vi "PathPlanner_PathPlanner_CreatePath.vi"(8 "Reversed":bool, 9 "MaxAcceleration":dbl, 10 "MaxVelocity":dbl, 11 "PathPlannerWayPoints":T7[](array[typedef]) {"HolonomicRotation"."SIN" format="%13.4f"; "HolonomicRotation"."COS" format="%13.4f"; "HolonomicRotation"."VALUE" format="%13.4f"; "NextControl"."Y" format="%14.3f"; "NextControl"."X" format="%14.3f"; "PrevControl"."Y" format="%14.3f"; "PrevControl"."X" format="%14.3f"; "AnchorPoint"."Y" format="%14.3f"; "AnchorPoint"."X" format="%14.3f"}) -> (3 "PathPlannerTrajectory":T1 {"States"."HolonomicRotation"."SIN" format="%13.4f"; "States"."HolonomicRotation"."COS" format="%13.4f"; "States"."HolonomicRotation"."VALUE" format="%13.4f"; "States"."AngularVelocity"."SIN" format="%13.4f"; "States"."AngularVelocity"."COS" format="%13.4f"; "States"."AngularVelocity"."VALUE" format="%13.4f"; "States"."TrajectoryState"."POSE"."ROTATION"."SIN" format="%13.4f"; "States"."TrajectoryState"."POSE"."ROTATION"."COS" format="%13.4f"; "States"."TrajectoryState"."POSE"."ROTATION"."VALUE" format="%13.4f"; "States"."TrajectoryState"."POSE"."TRANSLATION"."Y" format="%14.3f"; "States"."TrajectoryState"."POSE"."TRANSLATION"."X" format="%14.3f"; "States"."AngularAcceleration"."SIN" format="%13.4f"; "States"."AngularAcceleration"."COS" format="%13.4f"; "States"."AngularAcceleration"."VALUE" format="%13.4f"})   [LabVIEW 2019, in "PathPlanner.lvlib"]
doc: "Create a path from an array of PathPlanner Waypoints. This routine calculates the trajectory states. It handles combining separate paths when reversal is flagged.\n\nInputs:\n - PathPlannerWaypoints -- An array of PathPlannerWaypoints. This array must contain at least 2 entries.\n - maxVel -- Max velocity of the path\n - maxAccel -- Max velocity of the path\n - reversed -- Should the robot follow the path reversed\n\nOutputs:\n - PathPlanner Trajectory -- The generated path (path planner trajectory) can be converted to trajectory)"
uses:
  PathPlanner.lvlib
  <vilib>/Rock Robotics/WPI/ThirdParty/JAS_Junk/TrajLib/TRANSLATION2D.ctl
  <vilib>/Rock Robotics/WPI/ThirdParty/JAS_Junk/TrajLib/Trajectory_Library.lvlib
  <vilib>/Rock Robotics/WPI/ThirdParty/JAS_Junk/TrajLib/ROTATION2D.ctl
  PathPlannerWaypoint.ctl
  <vilib>/Rock Robotics/WPI/ThirdParty/JAS_Junk/TrajLib/POSE2D.ctl
  <vilib>/Rock Robotics/WPI/ThirdParty/JAS_Junk/TrajLib/TRAJ_STATE.ctl
  PathPlannerState.ctl
  PathPlannerTrajectory.ctl
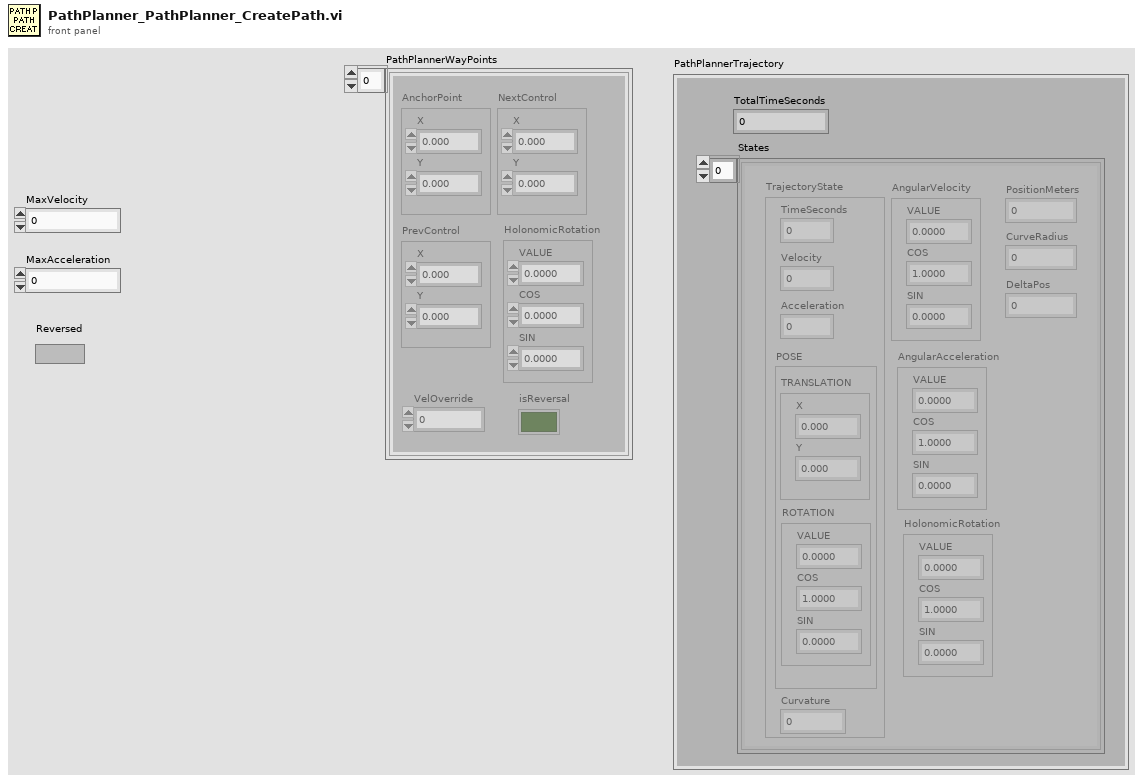
[diagram p1: front panel]
types:
  T1 = typedef "PathPlanner.lvlib/PathPlannerTrajectory.ctl" = cluster{"TotalTimeSeconds":dbl, "States":T2[]}
  T2 = typedef "PathPlanner.lvlib/PathPlannerState.ctl" = cluster{"AngularAcceleration":T3, "PositionMeters":dbl, "TrajectoryState":T4, "AngularVelocity":T3, "HolonomicRotation":T3, "CurveRadius":dbl, "DeltaPos":dbl}
  T3 = typedef "Trajectory_Library.lvlib/ROTATION2D.ctl" = cluster{"VALUE":dbl, "COS":dbl, "SIN":dbl}
  T4 = typedef "Trajectory_Library.lvlib/TRAJ_STATE.ctl" = cluster{"TimeSeconds":dbl, "Velocity":dbl, "Acceleration":dbl, "POSE":T5, "Curvature":dbl}
  T5 = typedef "Trajectory_Library.lvlib/POSE2D.ctl" = cluster{"TRANSLATION":T6, "ROTATION":T3}
  T6 = typedef "Trajectory_Library.lvlib/TRANSLATION2D.ctl" = cluster{"X":dbl, "Y":dbl}
  T7 = typedef "PathPlanner.lvlib/PathPlannerWaypoint.ctl" = cluster{"AnchorPoint":T6, "PrevControl":T6, "NextControl":T6, "HolonomicRotation":T3, "VelOverride":dbl, "isReversal":bool}
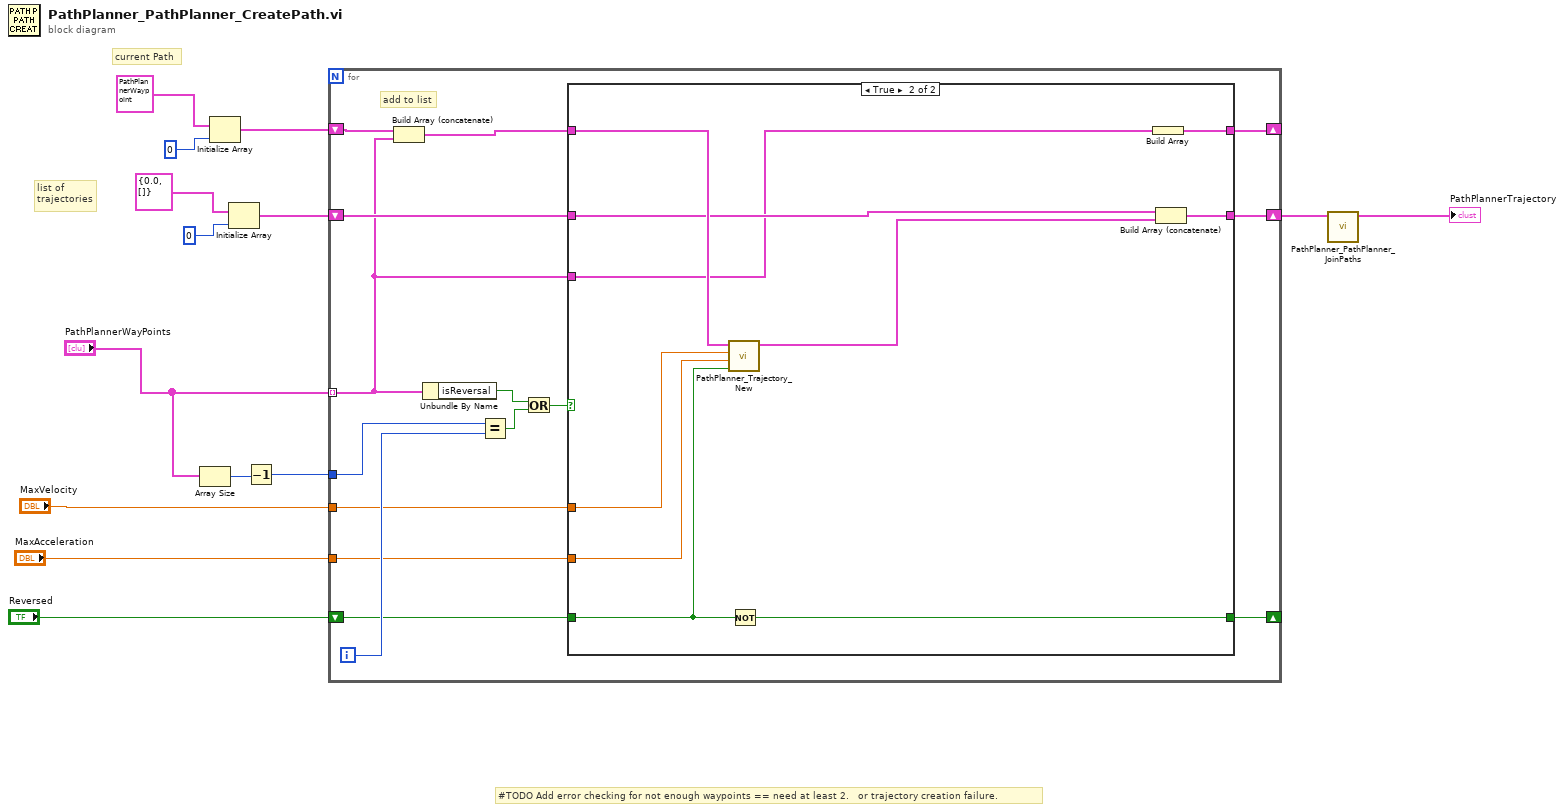
[diagram p0: block diagram]
diagram:
  # "#TODO Add error checking for not enough waypoints == need at least 2.   or trajectory creation failure."
  # "list of \ntrajectories"
  # "current Path"
  n1 = Array Size(array="PathPlannerWayPoints") -> (size(s)=w9:i32)
  n2 = Initialize Array(T7 {"AnchorPoint"={"X"=0.0, "Y"=0.0}, "PrevControl"={"X"=0.0, "Y"=0.0}, "NextControl"={"X"=0.0, "Y"=0.0}, "HolonomicRotation"={"VALUE"=0.0, "COS"=1.0, "SIN"=0.0}, "VelOverride"=0.0, "isReversal"=FALSE} ("PathPlannerWaypoint"), 0 ("dimension size")) -> (w12:T7[])
  n3 = Initialize Array(T1 {"TotalTimeSeconds"=0.0, "States"=[]} ("PathPlannerTrajectory"), 0 ("dimension size")) -> (w7:T1[])
  n4 = Decrement(x=w9) -> (x-1=w8:i32)
  n5 = for {
    shift-right: [w20] -> _
    shift-left: w12 -> [w29]
    tunnel: "PathPlannerWayPoints" -> [w15] mode=indexing
    tunnel: w8 -> [w26]
    shift-right: [w22] -> w1
    shift-left: w7 -> [w23]
    tunnel: "MaxVelocity" -> [w19]
    tunnel: "MaxAcceleration" -> [w18]
    shift-right: [w16] -> _
    shift-left: "Reversed" -> [w17]
    i -> [w25]
    # "add to list"
    n6 = Build Array (concatenate)(w29, w15) -> (w21:T7[])
    n7 = Unbundle By Name(w15) -> ("isReversal"=w28:bool)
    n8 = Equal?(x=w26, y=w25) -> (x = y?=w27:bool)
    n9 = Or(x=w28, y=w27) -> (x .or. y?=w24:bool)
    n10 = case shown="True" w24 {
      tunnel: w23 -> [w32 w38]
      tunnel: [w32 w39] -> w22
      tunnel: w21 -> [w31 w42]
      tunnel: [w31 w34] -> w20
      tunnel: w19 -> [_ w41]
      tunnel: w18 -> [_ w40]
      tunnel: w17 -> [w30 w35]
      tunnel: [w30 w36] -> w16
      tunnel: w15 -> [_ w33]
      frame False {
      }
      frame True {
        n11 = call "PathPlanner_Trajectory_New.vi"("Reversed"=w35, "MaxAccel"=w40, "MaxVelocity"=w41, "PathPoints"=w42) -> ("PathPlannerTrajectory"=w37:T1)  [unwired: 7 in]
        n12 = Not(x=w35) -> (.not. x?=w36:bool)
        n13 = Build Array(w33) -> (w34:T7[])
        n14 = Build Array (concatenate)(w38, w37) -> (w39:T1[])
      }
    }
  }
  n15 = call "PathPlanner_PathPlanner_JoinPaths.vi"("in Trajectories"=w1) -> ("out PathPlannerTrajectory"=→"PathPlannerTrajectory":T1)  [unwired: 10 in]
